vi "MSScript_SubVI_BreakStringToParams.vi"(1 "string":cluster{"Str":string, "Start":i32}) -> (0 "PARAMs":cluster{"Str":string, "Start":i32}[](array[cluster]))   [LabVIEW 2018, in "MSScript.lvclass"]
uses:
  MSScript.lvclass
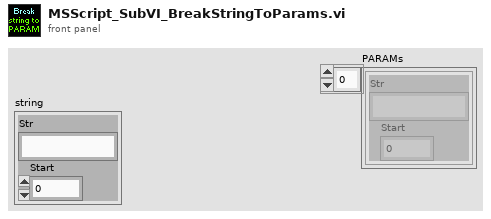
[diagram p1: front panel]
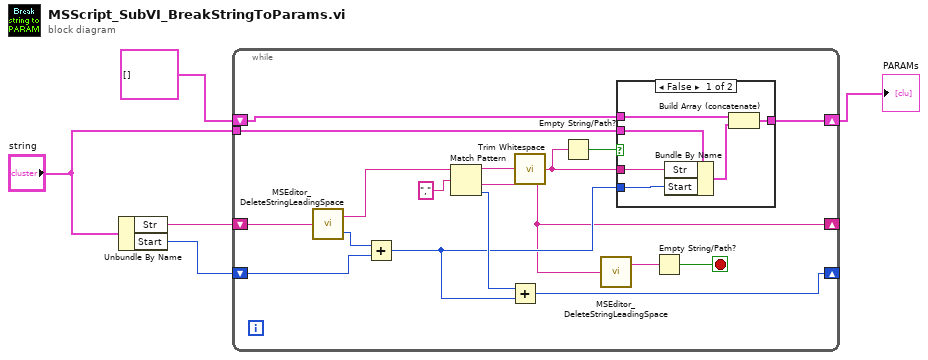
[diagram p0: block diagram]
diagram:
  n1 = Unbundle By Name("string") -> ("Str"=w5:string, "Start"=w4:i32)
  n2 = while {
    shift-right: [w10] -> _
    shift-left: w5 -> [w22]
    shift-right: [w13] -> _
    shift-left: w4 -> [w20]
    tunnel: "string" -> [w16]
    shift-right: [w7] -> w2
    shift-left: cluster{"Str":string, "Start":i32}[] [] -> [w6]
    stop <- w11 stop-if-true
    n3 = call "MSEditor_DeleteStringLeadingSpace.vi"("string in"=w22) -> ("string after leading space"=w19:string, "offset past leading space"=w21:i32)
    n4 = Add(x=w21, y=w20) -> (x+y=w14:i32)
    n5 = Match Pattern(string=w19, regular expression=",") -> (before substring=w15:string, after substring=w10:string, offset past match=w17:i32)  [unwired: 1 in, 1 out]
    n6 = Add(x=w17, y=w14) -> (x+y=w13:i32)
    n7 = call <vilib>:"Trim Whitespace.vi"("string"=w15) -> ("trimmed string"=w9:string)  [unwired: 1 in]
    n8 = Empty String/Path?(string/path=w9) -> (empty?=w8:bool)
    n9 = call "MSEditor_DeleteStringLeadingSpace.vi"("string in"=w10) -> ("string after leading space"=w12:string)  [unwired: 1 out]
    n10 = case shown="False" w8 {
      tunnel: w16 -> [w28 _]
      tunnel: w14 -> [w27 _]
      tunnel: w9 -> [w26 _]
      tunnel: [w24 w29] -> w7
      tunnel: w6 -> [w23 w29]
      frame False {
        n11 = Bundle By Name(cluster=w28, "Str"=w26, "Start"=w27) -> (w25:cluster{"Str":string, "Start":i32})
        n12 = Build Array (concatenate)(w23, w25) -> (w24:cluster{"Str":string, "Start":i32}[])
      }
      frame True {
      }
    }
    n13 = Empty String/Path?(string/path=w12) -> (empty?=w11:bool)
  }
  "PARAMs" <- w2
